vi "VBattSense SPI Test.vi"() -> ()   [LabVIEW 2011]
uses:
  TestCode/spiTest/FPGA/Controls/FPGA SPI_Communication Loop State.ctl
  TestCode/spiTest/FPGA/Controls/Port Action.ctl
  <vilib>/Platform/TimedLoop/XDataNode/wakeup.ctl
  <vilib>/Platform/TimedLoop/XDataNode/XDNodeRunTimeDep.lvlib
  <vilib>/Platform/TimedLoop/XDataNode/nitl_modes.ctl
  <vilib>/Platform/TimedLoop/XDataNode/timing_clust.ctl
  <vilib>/Platform/TimedLoop/XDataNode/XDataNode.xnode
  <vilib>/eio/EIONode/EIONode.xnode
  <vilib>/rvi/eio/common/nirviEmuTemplateMethod_errors.vi
panel:
  out "Battery Voltage":bool[](array[boolean])
  in  "Wait Ticks":u32=2000
  in  "SPI_Read":bool
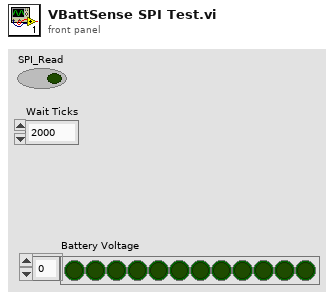
[diagram p1: front panel]
types:
  T1 = typedef "FPGA SPI_Communication Loop State.ctl" = enum8{"Idle", "Read"}
  T2 = typedef "Port Action.ctl" = enum8{"Start Read", "Transition", "Wait Cycles", "End Read"}
  T3 = typedef "XDNodeRunTimeDep.lvlib/timing_clust.ctl" = cluster{"Expected End [f-1]":u64, "Actual End [f-1]":u64, "Finished Late? [f-1]":bool, "Expected End [i-1]":u64, "Actual End [i-1]":u64, "Finished Late? [i-1]":bool, "Expected Start [i]":u64, "Actual Start [i]":u64, "Expected Start [f]":u64, "Actual Start [f]":u64, "Source Name":string, "Structure Name":string, "Period":i64, "Deadline":i64, "Offset":i64, "Start":i64, "Priority":i32, "Timeout":i32, "Mode":T4, "Wakeup Reason":T5, "Error":errorcluster, "Source Type":string, "Secondary Source Type":string, "Global End Time":u64, "Global Start Time":u64, "Frame Duration":u64, "Iteration Duration":u64, "Assigned CPU":i32, "I/O Scan Engine Mode":u32}
  T4 = typedef "XDNodeRunTimeDep.lvlib/nitl_modes.ctl" = enum32{"No Change", "Process missed periods, maintain original phase", "Discard missed periods, maintain original phase", "Process missed periods, ignore original phase", "Discard missed periods, ignore original phase"}
  T5 = typedef "XDNodeRunTimeDep.lvlib/wakeup.ctl" = enum32{"Normal", "Aborted", "Asynchronous wakeup", "Timing source error", "Timed loop error", "Timeout"}
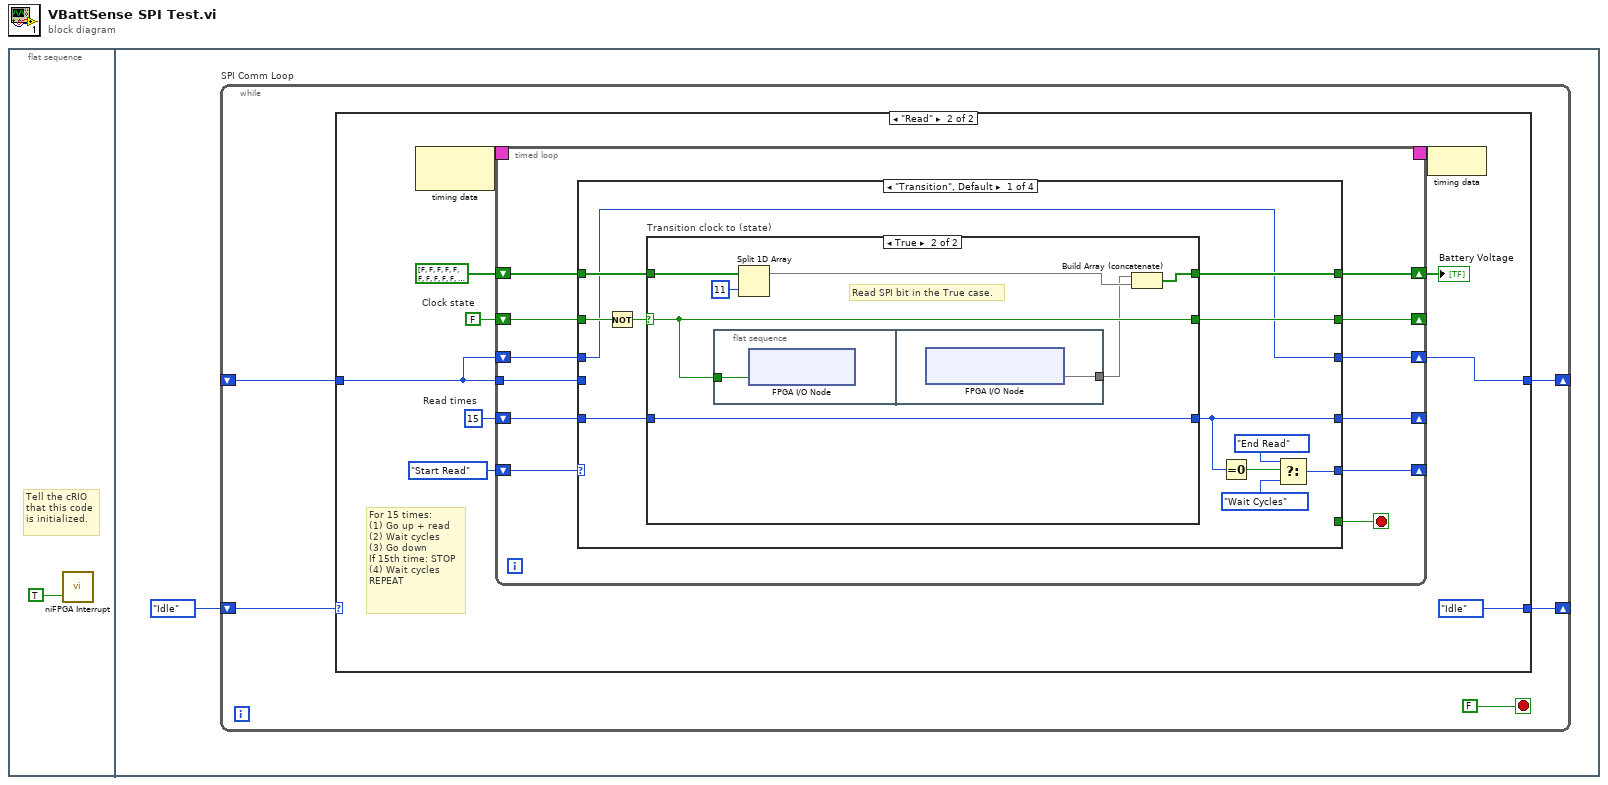
[diagram p0: block diagram]
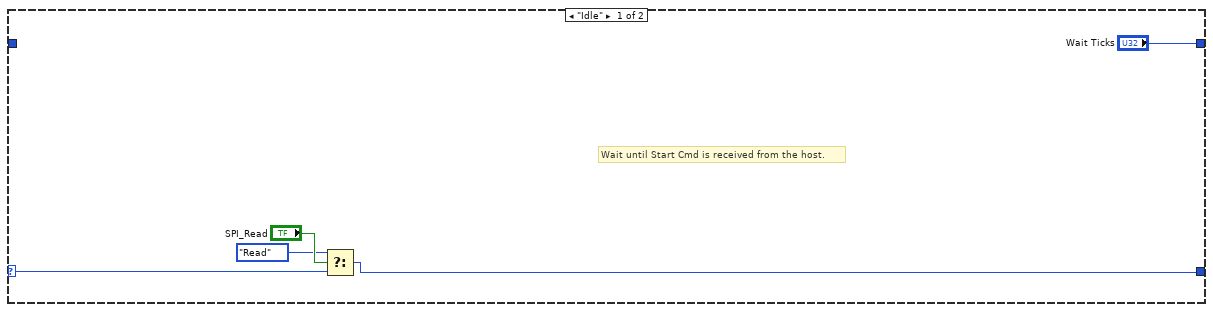
[diagram p2: hidden frame]
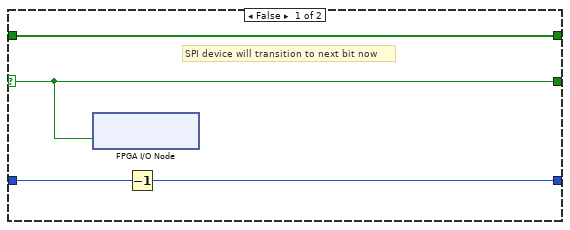
[diagram p3: hidden frame]
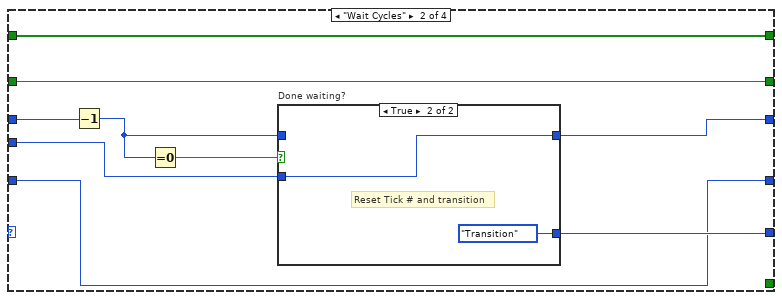
[diagram p4: hidden frame]
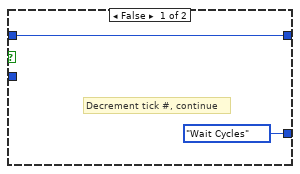
[diagram p5: hidden frame]
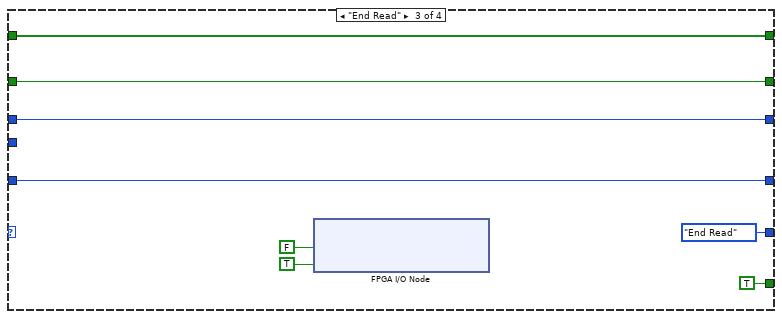
[diagram p6: hidden frame]
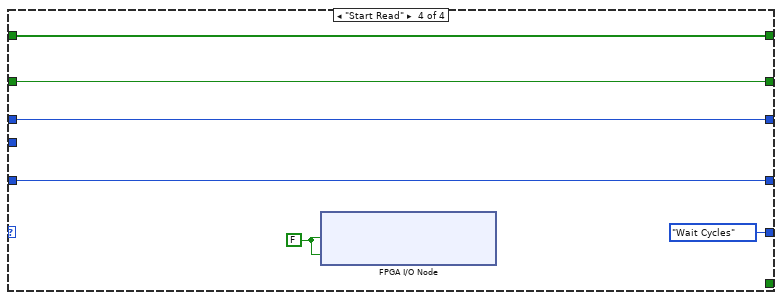
[diagram p7: hidden frame]
diagram:
  n1 = flat-sequence {
    frame #0 {
      # "Tell the cRIO\nthat this code\nis initialized."
      n2 = call <vilib>:"niFPGA Interrupt.vi"("Wait Until Cleared"=TRUE) -> ()  [unwired: 2 in]
    }
    frame #1 {
      n3 = while "SPI Comm Loop" {
        shift-right: [w6] -> _
        shift-left: FPGA_SPI_Communication_Loop_State."Idle" ("Action") -> [w5]
        shift-right: [w3] -> _
        shift-left: _ -> [w4]
        stop <- FALSE stop-if-true
        n4 = case shown="\"Read\"" w5 {
          selector: w5 -> [w11 _]
          tunnel: [w9 FPGA_SPI_Communication_Loop_State."Idle" ("Action")] -> w6
          tunnel: w4 -> [_ w14]
          tunnel: ["Wait Ticks" w13] -> w3
          frame "Idle" {
            # "Wait until Start Cmd is received from the host."
            n5 = Select(t=FPGA_SPI_Communication_Loop_State."Read" ("Action"), s="SPI_Read", f=w11) -> (s? t:f=w9:T1)
          }
          frame "Read" {
            w15 = FALSE  # Clock state
            w16 = u8 15  # Read times
            # "For 15 times:\n(1) Go up + read\n(2) Wait cycles\n(3) Go down\nIf 15th time: STOP\n(4) Wait cycles\nREPEAT"
            n6 = node-c288() -> (w21:T3)  [unwired: 1 out]
            n7 = timed-loop {
              timing-out: [_] -> w20
              timing: w21 -> [_]
              shift-right: [w27] -> _
              shift-left: Port_Action."Start Read" ("Action") -> [w34]
              shift-right: [w30] -> w17
              shift-left: bool[] [FALSE, FALSE, FALSE, FALSE, FALSE, FALSE, FALSE, FALSE, FALSE, FALSE, FALSE, FALSE] ("Battery Voltage") -> [w31]
              shift-right: [w32] -> _
              shift-left: w15 -> [w33]
              tunnel: w14 -> [w25]
              shift-right: [w24] -> w13
              shift-left: w14 -> [w26]
              shift-right: [w28] -> _
              shift-left: w16 -> [w29]
              stop <- w23 stop-if-true
              n8 = case shown="\"Transition\", Default" w34 {
                tunnel: w33 -> [w46 w68 w76 w84]
                tunnel: [w45 w68 w76 w84] -> w32
                tunnel: w31 -> [w43 w67 w75 w85]
                tunnel: [w42 w67 w75 w85] -> w30
                tunnel: w29 -> [w41 w60 w79 w82]
                tunnel: [w39 w60 w79 w82] -> w28
                tunnel: [w37 w63 Port_Action."End Read" ("Action") Port_Action."Wait Cycles" ("Action")] -> w27
                tunnel: w26 -> [w40 w66 w77 w83]
                tunnel: w25 -> [_ w61 _ _]
                tunnel: [w40 w62 w77 w83] -> w24
                tunnel: [_ _ TRUE _] -> w23
                frame "Transition", Default {
                  n9 = Not(x=w46) -> (.not. x?=w44:bool)
                  n10 = case "Transition clock to (state)" shown="True" w44 {
                    selector: w44 -> [w50 w57]
                    tunnel: [w50 w57] -> w45
                    tunnel: w43 -> [w47 w56]
                    tunnel: [w47 w54] -> w42
                    tunnel: w41 -> [w49 w53]
                    tunnel: [w48 w53] -> w39
                    frame False {
                      # "SPI device will transition to next bit now"
                      n11 = xnode "FPGA I/O Node"("VBatt_Clock"=w50) -> ()  [unwired: 1 in, 1 out]
                      n12 = Decrement(x=w49) -> (x-1=w48:u8)
                    }
                    frame True {
                      # "Read SPI bit in the True case."
                      n13 = flat-sequence {
                        tunnel: w57 -> [w58]
                        tunnel: [w59] -> w51
                        frame #0 {
                          n14 = xnode "FPGA I/O Node"("VBatt_Clock"=w58) -> ()  [unwired: 1 in, 1 out]
                        }
                        frame #1 {
                          n15 = xnode "FPGA I/O Node"() -> ("VBatt_DigitalInput"=w59)  [unwired: 1 in, 1 out]
                        }
                      }
                      n16 = Split 1D Array(array=w56, index=11) -> (first subarray=w52:bool[])  [unwired: 1 out]
                      n17 = Build Array (concatenate)(w51, w52) -> (w54:bool[])
                    }
                  }
                  n18 = Equal To 0?(x=w39) -> (x = 0?=w38:bool)
                  n19 = Select(t=Port_Action."End Read" ("Action"), s=w38, f=Port_Action."Wait Cycles" ("Action")) -> (s? t:f=w37:T2)
                }
                frame "Wait Cycles" {
                  n20 = Decrement(x=w66) -> (x-1=w64:u32)
                  n21 = Equal To 0?(x=w64) -> (x = 0?=w65:bool)
                  n22 = case "Done waiting?" shown="True" w65 {
                    tunnel: w64 -> [w69 _]
                    tunnel: [Port_Action."Wait Cycles" ("Action") Port_Action."Transition" ("Action")] -> w63
                    tunnel: [w69 w71] -> w62
                    tunnel: w61 -> [_ w71]
                    frame False {
                      # "Decrement tick #, continue"
                    }
                    frame True {
                      # "Reset Tick # and transition"
                    }
                  }
                }
                frame "End Read" {
                  n23 = xnode "FPGA I/O Node"("VBatt_Clock"=FALSE ("VBatt_ChipSelectInverted"), "VBatt_ChipSelectInverted"=TRUE) -> ()  [unwired: 2 in, 2 out]
                }
                frame "Start Read" {
                  w86 = FALSE ("VBatt_ChipSelectInverted")
                  n24 = xnode "FPGA I/O Node"("VBatt_Clock"=w86, "VBatt_ChipSelectInverted"=w86) -> ()  [unwired: 2 in, 2 out]
                }
              }
            }
            "Battery Voltage" <- w17
            n25 = node-c288(w20) -> ()
          }
        }
      }
    }
  }
